vi "Get Class From DVR.vi"(8 "error in (no error)":errorcluster, 11 "DVR IN":refnum<data-value>) -> (0 "error out":errorcluster, 2 "Class name":string, 3 "DVR OUT":refnum<data-value>)   [LabVIEW 2020, in "TX Speed.lvclass"]
uses:
  TX Speed.lvclass
  TX Speed.lvclass/TX Speed.ctl
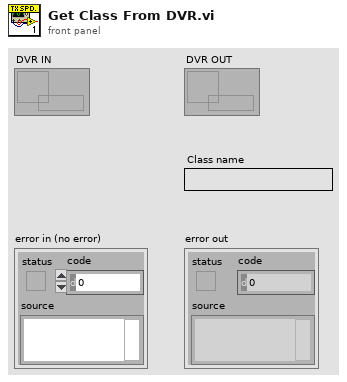
[diagram p1: front panel]
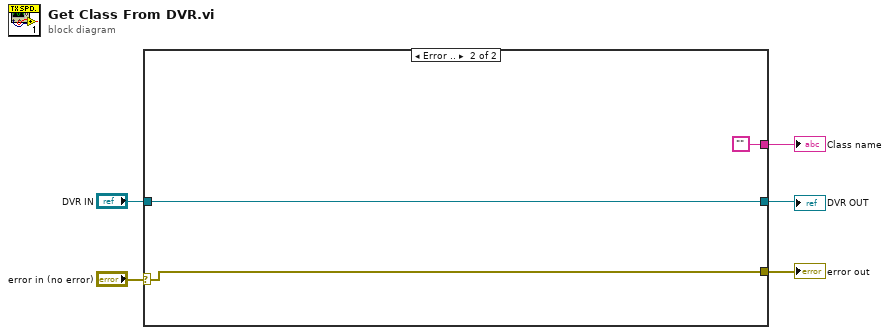
[diagram p0: block diagram]
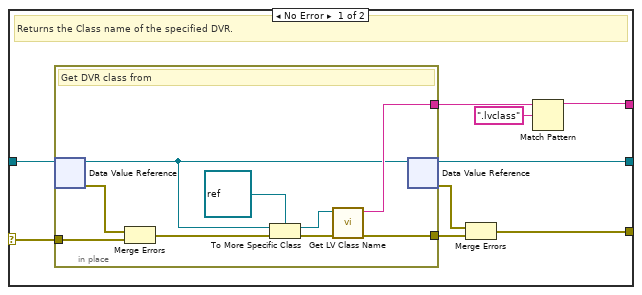
[diagram p2: hidden frame]
diagram:
  n1 = case shown="Error .." "error in (no error)" {
    selector: "error in (no error)" -> [w13 w25]
    tunnel: [w14 w24] -> w1
    tunnel: [w11 w25] -> w4
    tunnel: [w7 ""] -> w3
    tunnel: "DVR IN" -> [w6 w24]
    frame No Error {
      # "Returns the Class name of the specified DVR."
      n2 = in-place {
        in-place-border: w13 -> [w23]
        in-place-border: [w20] -> w10
        in-place-border: [w16] -> w9
        # "Get DVR class from"
        n3 = in-place-dvr #1(w6) -> (w15:refnum<class "TX Speed.lvclass">, w22:errorcluster)
        n4 = Merge Errors(w22, w23) -> (w21:errorcluster)
        n5 = To More Specific Class(target class=refnum<class> refnum ("LabVIEW Object"), reference=w15, error in=w21) -> (specific class reference=w17:refnum<class>, error out=w19:errorcluster)
        n6 = call <vilib>:"Get LV Class Name.vi"("error in (no error)"=w19, "object"=w17) -> ("error out"=w20:errorcluster, "class name"=w16:string)  [unwired: 8 in]
        n7 = in-place-dvr #1(w15) -> (w14:refnum<data-value>, w12:errorcluster)
      }
      n8 = Merge Errors(w12, w10) -> (w11:errorcluster)
      n9 = Match Pattern(string=w9, regular expression=".lvclass") -> (before substring=w7:string)  [unwired: 1 in, 3 out]
    }
    frame Error {
    }
  }
  "error out" <- w4
  "Class name" <- w3
  "DVR OUT" <- w1
